vi "update.vi"(8 "error in":errorcluster, 10 "settings cluster":T2, 11 "FPGA VI ref":T1) -> (0 "error out":errorcluster)   [LabVIEW 2010]
uses:
  type definitions/settings_cluster.ctl
  common_typedefs/channels_cluster.ctl
  type definitions/gate_cluster.ctl
  common_typedefs/gate_parameters_cluster.ctl
  FPGA_VI_reference.ctl
  <vilib>/rvi/interface/nirviReadWriteControl/nirviReadWriteControl.xnode
  <vilib>/rvi/interface/common/niFpgaNodeNameForErrorReporting.ctl
  <vilib>/rvi/errors/niLvFpgaWhatHappensToTopLevelVI.ctl
  <vilib>/Utility/error.llb/Error Cluster From Error Code.vi
  <vilib>/rvi/errors/niLvFpgaAdjustHostInterfaceError.vi
  NiFpgaLv.dll
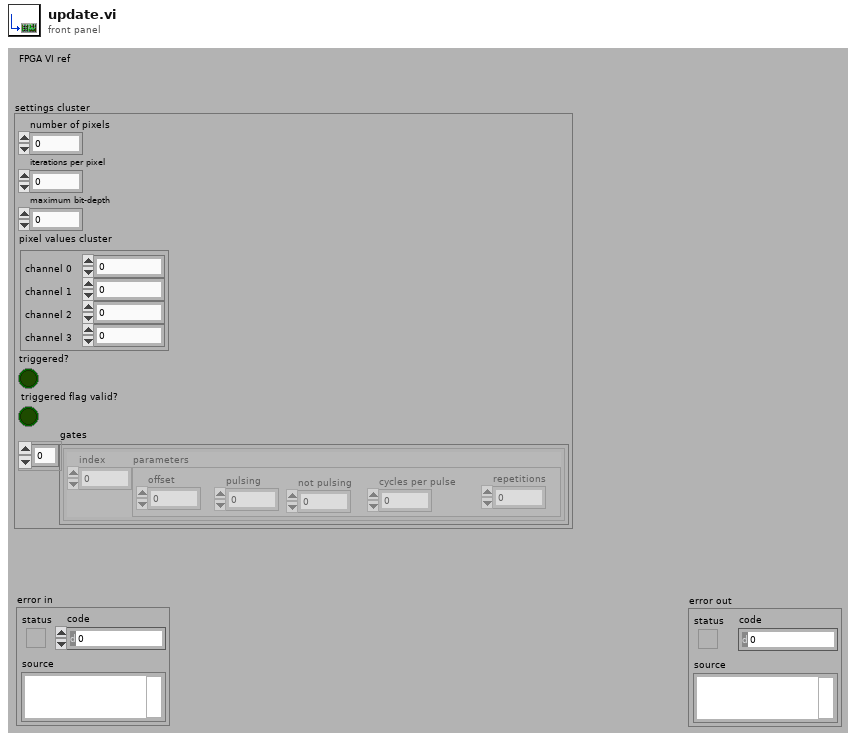
[diagram p1: front panel]
types:
  T1 = typedef "FPGA_VI_reference.ctl" = refnum<k20>
  T2 = typedef "settings_cluster.ctl" = cluster{"number of pixels":i32, "iterations per pixel":i32, "maximum bit-depth":i32, "pixel values cluster":T3, "triggered?":bool, "triggered flag valid?":bool, "gates":T4[]}
  T3 = typedef "channels_cluster.ctl" = cluster{"channel 0":u32, "channel 1":u32, "channel 2":u32, "channel 3":u32}
  T4 = typedef "gate_cluster.ctl" = cluster{"index":i32, "parameters":T5}
  T5 = typedef "gate_parameters_cluster.ctl" = cluster{"offset":i64, "pulsing":i64, "not pulsing":i64, "cycles per pulse":i64, "repetitions":i64}
  T6 = typedef "niFpgaNodeNameForErrorReporting.ctl" = enum16{"Open FPGA VI Reference", "Read/Write Control", "Invoke Method: Abort", "Invoke Method: Acknowledge IRQ", "Invoke Method: Download", "Invoke Method: FIFO.Configure", "Invoke Method: FIFO.Read", "Invoke Method: FIFO.Start", "Invoke Method: FIFO.Stop", "Invoke Method: FIFO.Write", "Invoke Method: Reset", "Invoke Method: Run", "Invoke Method: Wait on IRQ", "Close FPGA VI Reference"}
  T7 = typedef "niLvFpgaWhatHappensToTopLevelVI.ctl" = enum16{"top level VI scripted behind XNode", "top level VI inlined behind XNode"}
  T8 = cluster{"channel 0":u32, "channel 1":u32, "channel 2":u32, "channel 3":u32}
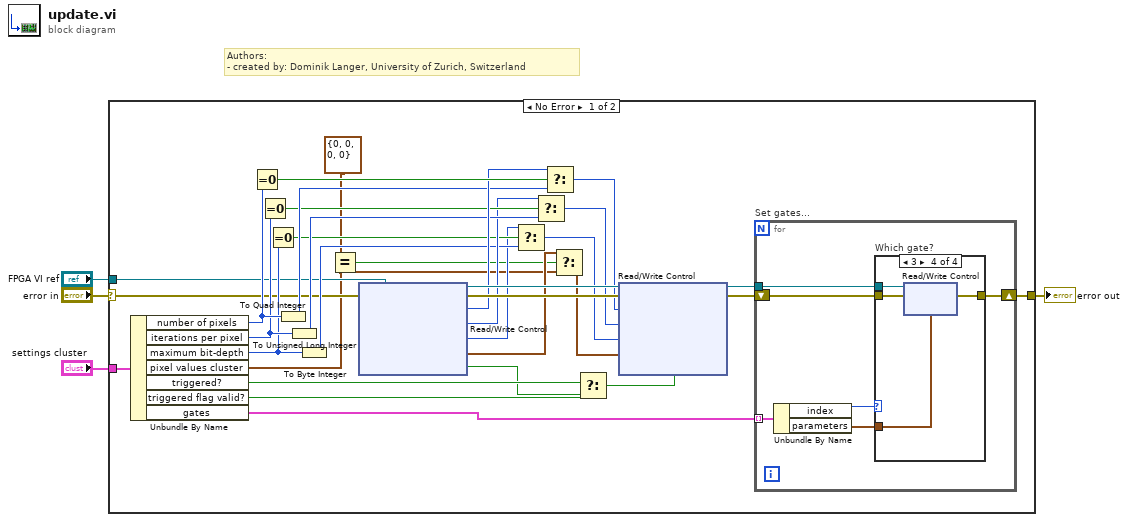
[diagram p0: block diagram]
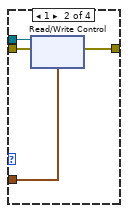
[diagram p3: hidden frame]
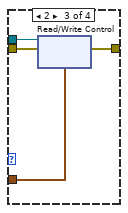
[diagram p4: hidden frame]
diagram:
  # "Authors: \n- created by: Dominik Langer, University of Zurich, Switzerland"
  n1 = case shown="No Error" "error in" {
    selector: "error in" -> [w16 w478]
    tunnel: "settings cluster" -> [w17 _]
    tunnel: [w6 w478] -> w2
    tunnel: "FPGA VI ref" -> [w15 _]
    frame No Error {
      n2 = Unbundle By Name(w17) -> ("number of pixels"=w35:i32, "iterations per pixel"=w30:i32, "maximum bit-depth"=w25:i32, "pixel values cluster"=w11:T3, "triggered?"=w19:bool, "triggered flag valid?"=w20:bool, "gates"=w8:T4[])
      n3 = Equal To 0?(x=w35) -> (x = 0?=w34:bool)
      n4 = Equal To 0?(x=w30) -> (x = 0?=w29:bool)
      n5 = Equal To 0?(x=w25) -> (x = 0?=w24:bool)
      n6 = To Quad Integer(1:w35) -> (0:w32:i64)
      n7 = To Unsigned Long Integer(number=w30) -> (unsigned 32bit integer=w28:u32)
      n8 = To Byte Integer(number=w25) -> (8bit integer=w23:i8)
      n9 = Equal?(x=T3 {"channel 0"=0, "channel 1"=0, "channel 2"=0, "channel 3"=0} ("pixel values cluster"), y=w11) -> (x = y?=w9:bool)
      n10 = xnode "Read/Write Control"("FPGA VI Reference In"=w15, "error in"=w16) -> ("FPGA VI Reference Out"=w37:T1, "error out"=w36:errorcluster, "number of pixels"=w33:i64, "iterations per pixel"=w27:u32, "maximum bit depth"=w22:i8, "channel offsets"=w13:T8, "wait for trigger?"=w14:bool)
      n11 = Select(t=w22, s=w24, f=w23) -> (s? t:f=w21:i8)
      n12 = Select(t=w27, s=w29, f=w28) -> (s? t:f=w26:u32)
      n13 = Select(t=w33, s=w34, f=w32) -> (s? t:f=w31:i64)
      n14 = Select(t=w13, s=w9, f=w11) -> (s? t:f=w12:T3)
      n15 = Select(t=w19, s=w20, f=w14) -> (s? t:f=w18:bool)
      n16 = xnode "Read/Write Control"("FPGA VI Reference In"=w37, "error in"=w36, "number of pixels"=w31, "iterations per pixel"=w26, "maximum bit depth"=w21, "channel offsets"=w12, "wait for trigger?"=w18) -> ("FPGA VI Reference Out"=w5:T1, "error out"=w7:errorcluster)
      n17 = for "Set gates..." {
        tunnel: w8 -> [w43] mode=indexing
        shift-right: [w39] -> w6
        shift-left: w7 -> [w42]
        tunnel: w5 -> [w41]
        n18 = Unbundle By Name(w43) -> ("index"=w40:i32, "parameters"=w38:T5)
        n19 = case "Which gate?" shown="3" w40 {
          tunnel: w42 -> [w44 w48 w94 w142]
          tunnel: w41 -> [_ w47 w96 w143]
          tunnel: [w44 w46 w93 w141] -> w39
          tunnel: w38 -> [_ w45 w95 w144]
          frame Default {
          }
          frame 1 {
            n20 = xnode "Read/Write Control"("FPGA VI Reference In"=w47, "error in"=w48, "gate 1"=w45) -> ("error out"=w46:errorcluster)  [unwired: 1 out]
          }
          frame 2 {
            n21 = xnode "Read/Write Control"("FPGA VI Reference In"=w96, "error in"=w94, "gate 2"=w95) -> ("error out"=w93:errorcluster)  [unwired: 1 out]
          }
          frame 3 {
            n22 = xnode "Read/Write Control"("FPGA VI Reference In"=w143, "error in"=w142, "gate 3"=w144) -> ("error out"=w141:errorcluster)  [unwired: 1 out]
          }
        }
      }
    }
    frame Error {
    }
  }
  "error out" <- w2
